vi "-Parse_Authentication_Response.vi"(8 "error in (no error)":errorcluster, 11 "Postgres Connector In":refnum<class "Postgres Connector.lvclass">) -> (0 "error out":errorcluster, 3 "Postgres Connector Out":refnum<class "Postgres Connector.lvclass">)   [LabVIEW 2019, in "PG_LIB.lvlib" / "Postgres Connector.lvclass"]
doc: "This VI is used to filter the response of the database. Depending of the type of authentication recquired, the good case will be choosen and therefore the good method of authentication."
uses:
  Postgres Connector.lvclass
  Postgres Connector.lvclass/Postgres Connector.ctl
  hashlib/hashlib/hashlib.lvlib
panel:
  out "Answer From Server":string
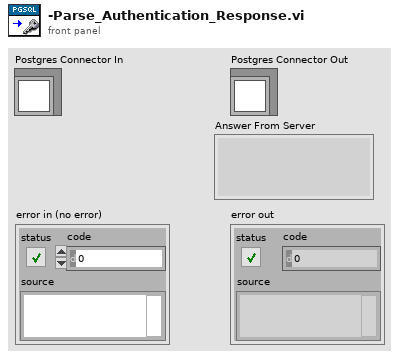
[diagram p1: front panel]
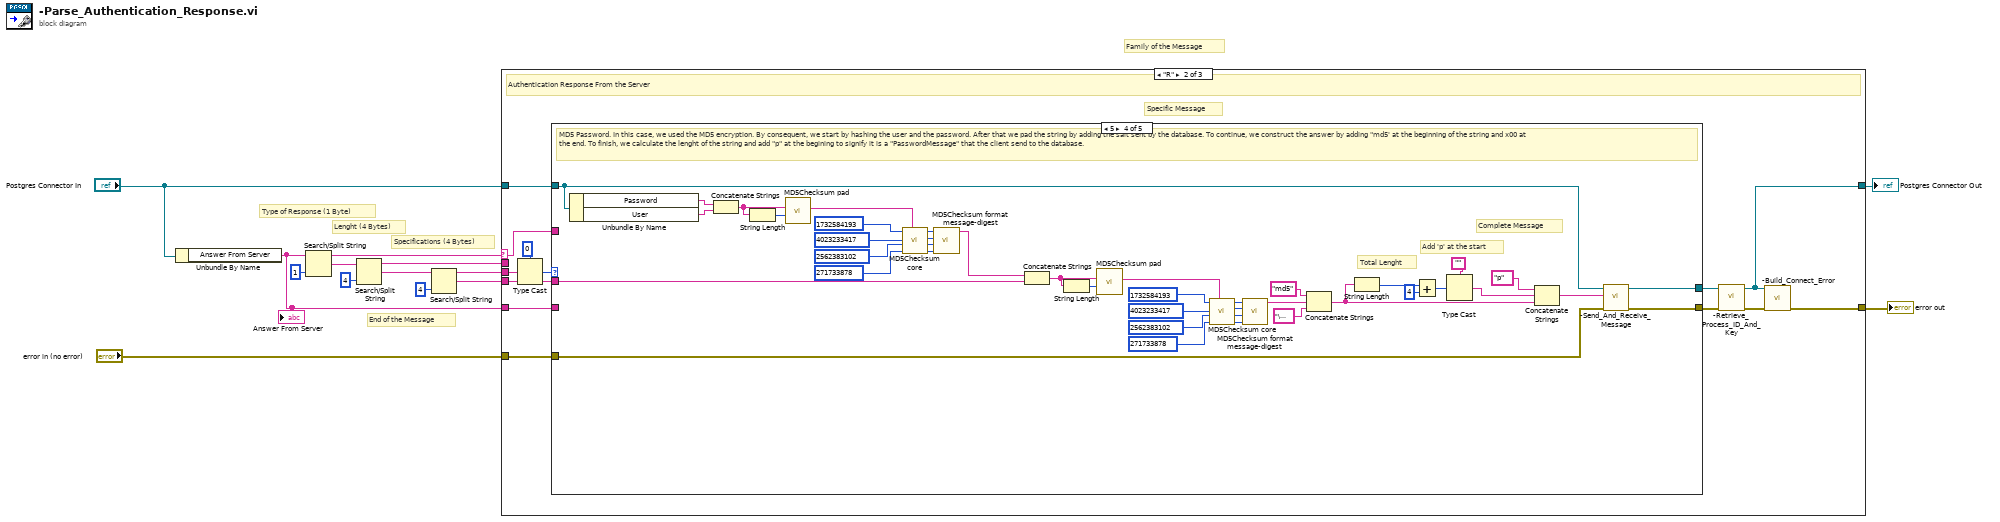
[diagram p0: block diagram]
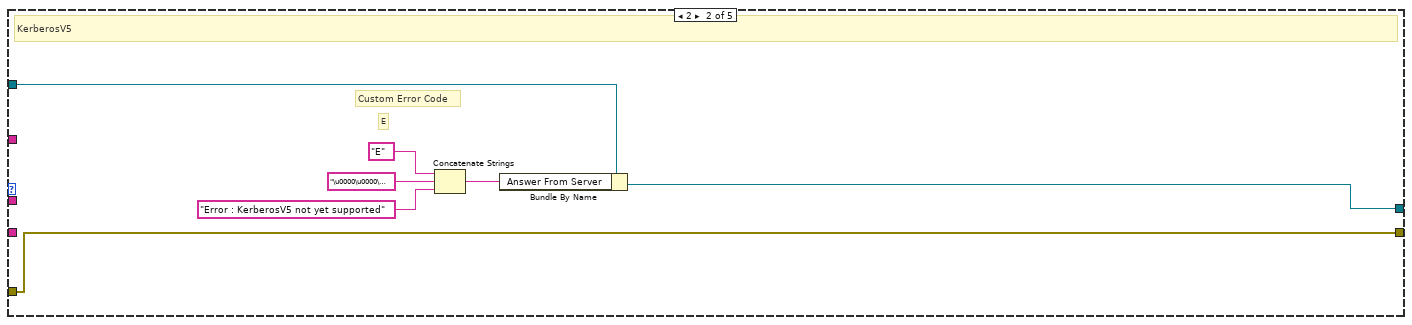
[diagram p4: hidden frame]
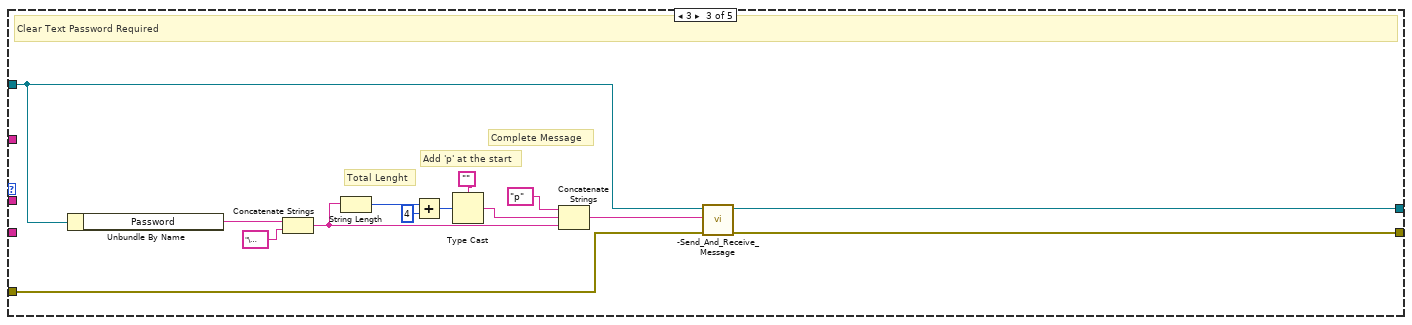
[diagram p5: hidden frame]
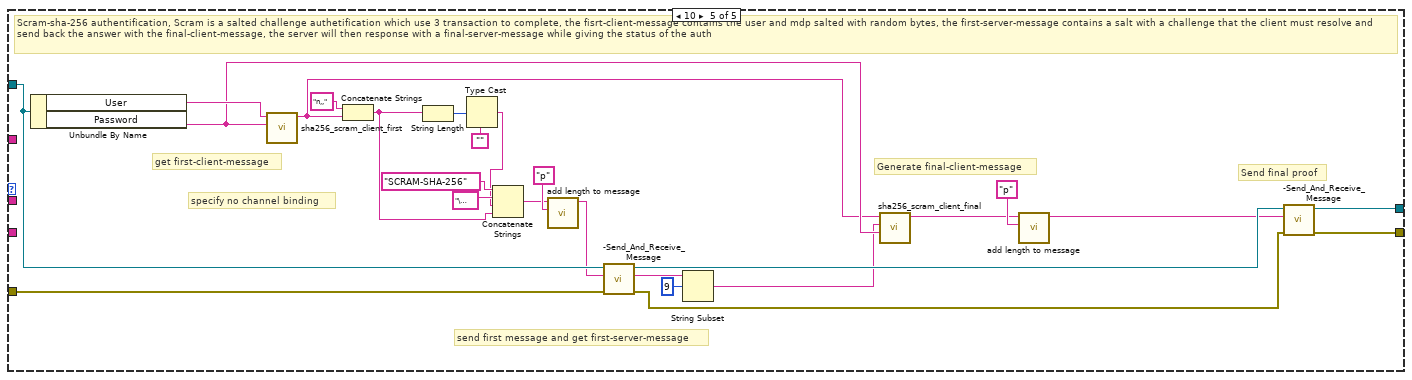
[diagram p6: hidden frame]
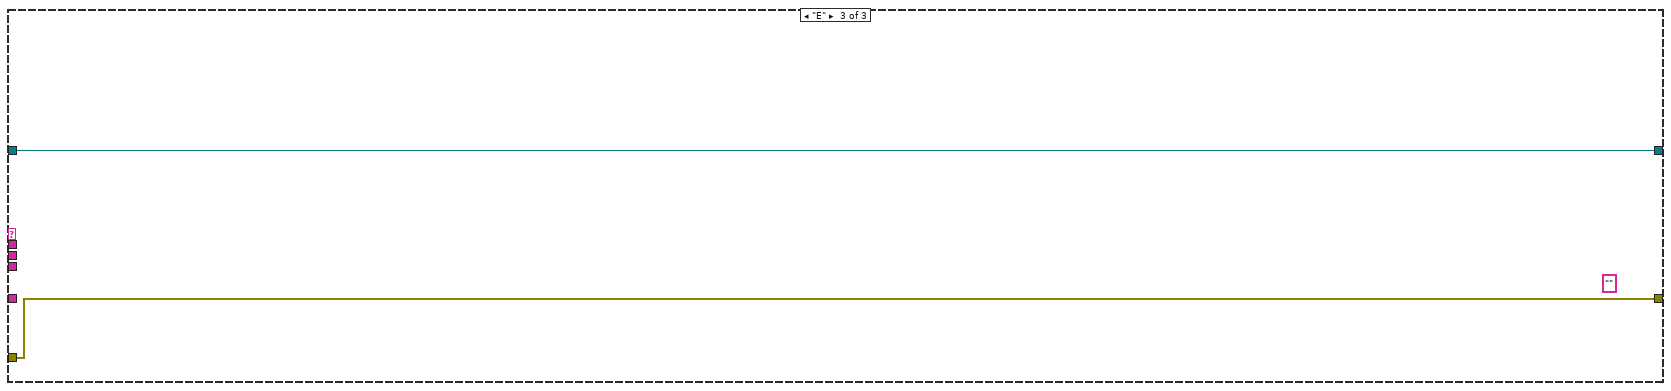
[diagram p7: hidden frame]
diagram:
  # "Family of the Message"
  # "End of the Message"
  # "Specifications (4 Bytes)"
  # "Lenght (4 Bytes)"
  # "Type of Response (1 Byte)"
  n1 = Unbundle By Name("Postgres Connector In") -> ("Answer From Server"=w1:string)
  "Answer From Server" <- w1
  n2 = Search/Split String(string=w1, offset (0)=1 ("length (rest)")) -> (substring before match=w11:string, match + rest of string=w10:string)  [unwired: 1 in, 1 out]
  n3 = Search/Split String(string=w10, offset (0)=4 ("length (rest)")) -> (substring before match=w6:string, match + rest of string=w9:string)  [unwired: 1 in, 1 out]
  n4 = Search/Split String(string=w9, offset (0)=4 ("length (rest)")) -> (substring before match=w8:string, match + rest of string=w7:string)  [unwired: 1 in, 1 out]
  n5 = case shown="\"R\"" w11 {
    selector: w11 -> [_ w23 _]
    tunnel: w8 -> [_ w29 _]
    tunnel: w7 -> [_ w26 _]
    tunnel: w6 -> [_ _ _]
    tunnel: "Postgres Connector In" -> [w15 w25 w119]
    tunnel: [w16 w22 w120] -> w5
    tunnel: "error in (no error)" -> [w16 w24 w120]
    tunnel: [w15 w18 w119] -> w2
    tunnel: w1 -> [_ w17 _]
    frame "0", Default {
    }
    frame "R" {
      # "Specific Message"
      # "Authentication Response From the Server"
      n6 = Type Cast(type=0, x=w29) -> (*(type *) &x=w27:i32)
      n7 = case shown="5" w27 {
        tunnel: w26 -> [_ _ _ w61 _]
        tunnel: w25 -> [w30 w37 w41 w59 w112]
        tunnel: [w31 w38 w39 w56 w117] -> w21
        tunnel: w24 -> [w31 w38 w43 w58 w106]
        tunnel: w23 -> [_ _ _ _ _]
        tunnel: [w30 w35 w40 w57 w118] -> w20
        tunnel: w17 -> [_ _ _ _ _]
        frame 0, Default {
          # "Authentication OK"
        }
        frame 2 {
          # "Custom Error Code"
          # "E"
          # "KerberosV5"
          n8 = Concatenate Strings("E" ("Answer From Server"), "\u0000\u0000\u0000\u0000" ("Answer From Server"), "Error : KerberosV5 not yet supported" ("string")) -> (w34:string)
          n9 = Bundle By Name(cluster=w37, "Answer From Server"=w34) -> (w35:refnum<class "Postgres Connector.lvclass">)
        }
        frame 3 {
          # "Complete Message"
          # "Total Lenght"
          # "Add 'p' at the start"
          # "Clear Text Password Required"
          n10 = Unbundle By Name(w41) -> ("Password"=w44:string)
          n11 = Concatenate Strings(w44, "\u0000" ("string")) -> (w46:string)
          n12 = String Length(string=w46) -> (length=w51:i32)
          n13 = Add(x=w51, y=4) -> (x+y=w49:i32)
          n14 = Type Cast(type="", x=w49) -> (*(type *) &x=w52:string)
          n15 = Concatenate Strings("p", w52, w46) -> (w42:string)
          n16 = call "-Send_And_Receive_Message.vi"("error in (no error)"=w43, "Message To Send"=w42, "Postgres Connector In"=w41) -> ("error out"=w39:errorcluster, "Postgres Connector Out"=w40:refnum<class "Postgres Connector.lvclass">)  [unwired: 6 in, 1 out]
        }
        frame 5 {
          # "Complete Message"
          # "Total Lenght"
          # "Add 'p' at the start"
          # "MD5 Password. In this case, we used the MD5 encryption. By consequent, we start by hashing the user and the password. After that we pad the string by adding the salt sent by the database. To continue, we construct the answer by adding \"md5' at the beginning of the string and x00 at the end. To finish, we calculate the lenght of the string and add \"p\" at the begining to signify it is a \"PasswordMessage\" that the client send to the database."
          n17 = Unbundle By Name(w59) -> ("Password"=w53:string, "User"=w54:string)
          n18 = Concatenate Strings(w53, w54) -> (w78:string)
          n19 = String Length(string=w78) -> (length=w77:i32)
          n20 = call <vilib>:"MD5Checksum pad.vi"("Message String Length (bytes)"=w77, "Last Part of Message String"=w78) -> ("Padding"=w79:string)  [unwired: 9 in]
          n21 = call <vilib>:"MD5Checksum core.vi"("Input String"=w79, "s4 in"=u32 271733878 ("s4"), "s3 in"=u32 2562383102 ("s3"), "s2 in"=u32 4023233417 ("s2"), "s1 in"=u32 1732584193 ("s1")) -> ("s4 out"=w90:u32, "s3 out"=w91:u32, "s2 out"=w92:u32, "s1 out"=w93:u32)  [unwired: 3 in]
          n22 = call <vilib>:"MD5Checksum format message-digest.vi"("s4"=w90, "s3"=w91, "s2"=w92, "s1"=w93) -> ("MD5 message-digest"=w65:string)  [unwired: 7 in]
          n23 = Concatenate Strings(w65, w61) -> (w66:string)
          n24 = String Length(string=w66) -> (length=w76:i32)
          n25 = call <vilib>:"MD5Checksum pad.vi"("Message String Length (bytes)"=w76, "Last Part of Message String"=w66) -> ("Padding"=w75:string)  [unwired: 9 in]
          n26 = call <vilib>:"MD5Checksum core.vi"("Input String"=w75, "s4 in"=u32 271733878 ("s4"), "s3 in"=u32 2562383102 ("s3"), "s2 in"=u32 4023233417 ("s2"), "s1 in"=u32 1732584193 ("s1")) -> ("s4 out"=w70:u32, "s3 out"=w69:u32, "s2 out"=w68:u32, "s1 out"=w67:u32)  [unwired: 3 in]
          n27 = call <vilib>:"MD5Checksum format message-digest.vi"("s4"=w70, "s3"=w69, "s2"=w68, "s1"=w67) -> ("MD5 message-digest"=w64:string)  [unwired: 7 in]
          n28 = Concatenate Strings("md5" ("string"), w64, "\u0000" ("string")) -> (w63:string)
          n29 = String Length(string=w63) -> (length=w84:i32)
          n30 = Add(x=w84, y=4) -> (x+y=w82:i32)
          n31 = Type Cast(type="", x=w82) -> (*(type *) &x=w85:string)
          n32 = Concatenate Strings("p", w85, w63) -> (w60:string)
          n33 = call "-Send_And_Receive_Message.vi"("error in (no error)"=w58, "Message To Send"=w60, "Postgres Connector In"=w59) -> ("error out"=w56:errorcluster, "Postgres Connector Out"=w57:refnum<class "Postgres Connector.lvclass">)  [unwired: 6 in, 1 out]
        }
        frame 10 {
          # "Send final proof"
          # "send first message and get first-server-message"
          # "Generate final-client-message"
          # "specify no channel binding"
          # "get first-client-message"
          # "Scram-sha-256 authentification, Scram is a salted challenge authetification which use 3 transaction to complete, the fisrt-client-message contains the user and mdp salted with random bytes, the first-server-message contains a salt with a challenge that the client must resolve and send back the answer with the final-client-message, the server will then response with a final-server-message while giving the status of the auth"
          n34 = Unbundle By Name(w112) -> ("User"=w116:string, "Password"=w98:string)
          n35 = call "sha256_scram_client_first.vi"("password"=w98, "user"=w116) -> ("client_first_message"=w97:string)  [unwired: 9 in]
          n36 = Concatenate Strings("n,," ("string"), w97) -> (w95:string)
          n37 = String Length(string=w95) -> (length=w113:i32)
          n38 = Type Cast(type="", x=w113) -> (*(type *) &x=w108:string)
          n39 = Concatenate Strings("SCRAM-SHA-256" ("string"), "\u0000" ("string"), w108, w95) -> (w99:string)
          n40 = call "add length to message.vi"("header byte"="p", "message"=w99) -> ("message out"=w107:string)  [unwired: 9 in]
          n41 = call "-Send_And_Receive_Message.vi"("error in (no error)"=w106, "Message To Send"=w107, "Postgres Connector In"=w112) -> ("error out"=w103:errorcluster, "data out"=w105:string, "Postgres Connector Out"=w102:refnum<class "Postgres Connector.lvclass">)  [unwired: 6 in]
          n42 = String Subset(string=w105, offset (0)=9) -> (substring=w96:string)  [unwired: 1 in]
          n43 = call "sha256_scram_client_final.vi"("password"=w98, "server_first_message"=w96, "client_first_message"=w97) -> ("client_final_message"=w94:string)  [unwired: 8 in]
          n44 = call "add length to message.vi"("header byte"="p", "message"=w94) -> ("message out"=w100:string)  [unwired: 9 in]
          n45 = call "-Send_And_Receive_Message.vi"("error in (no error)"=w103, "Message To Send"=w100, "Postgres Connector In"=w102) -> ("error out"=w117:errorcluster, "Postgres Connector Out"=w118:refnum<class "Postgres Connector.lvclass">)  [unwired: 6 in, 1 out]
        }
      }
      n46 = call "-Retrieve_Process_ID_And_Key.vi"("error in (no error)"=w21, "Postgres Connector In"=w20) -> ("error out"=w19:errorcluster, "Postgres Connector Out"=w18:refnum<class "Postgres Connector.lvclass">)  [unwired: 8 in]
      n47 = call "-Build_Connect_Error.vi"("error in (no error)"=w19, "Postgres Connector In"=w18) -> ("error out"=w22:errorcluster)  [unwired: 9 in]
    }
    frame "E" {
      (unwired) "" ("Answer From Server")
    }
  }
  "error out" <- w5
  "Postgres Connector Out" <- w2
